vi "Temperature serial v7.vi"(0 "Command String":string, 5 "Time Out (S)":dbl, 7 "CALIB":dbl) -> (4 "T1":dbl, 6 "T2":dbl, 8 "T3":dbl, 10 "T4":dbl, 13 "error":bool, 14 "output cluster":cluster{dbl, dbl, dbl, dbl, i32, "error #":dbl}, 15 "Unit ID":dbl)   [LabVIEW 2017]
uses:
  Global 1.vi
panel:
  out "error out":errorcluster
  out "COM port":refnum<visa-resource-name>="COM6"
  out "error #":dbl
  out "End T":dbl
  out "Start T":dbl
  out "read time":dbl
  in  "Array - String":string[](array[string])
  out "end of data (#)":bool
  out "data bytes read":dbl
  out "data string":string
  out "read buffer":string
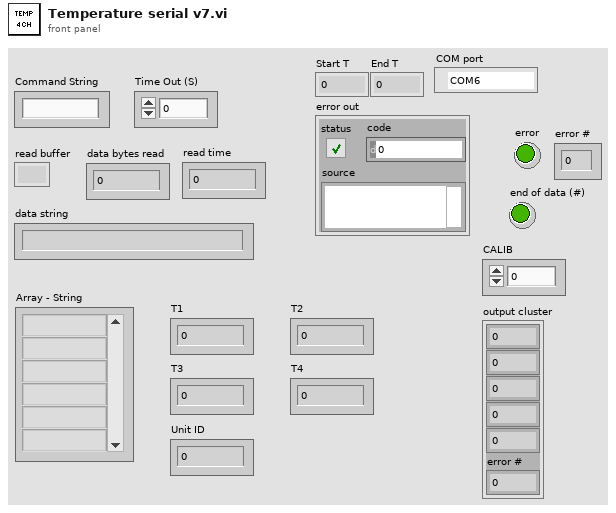
[diagram p1: front panel]
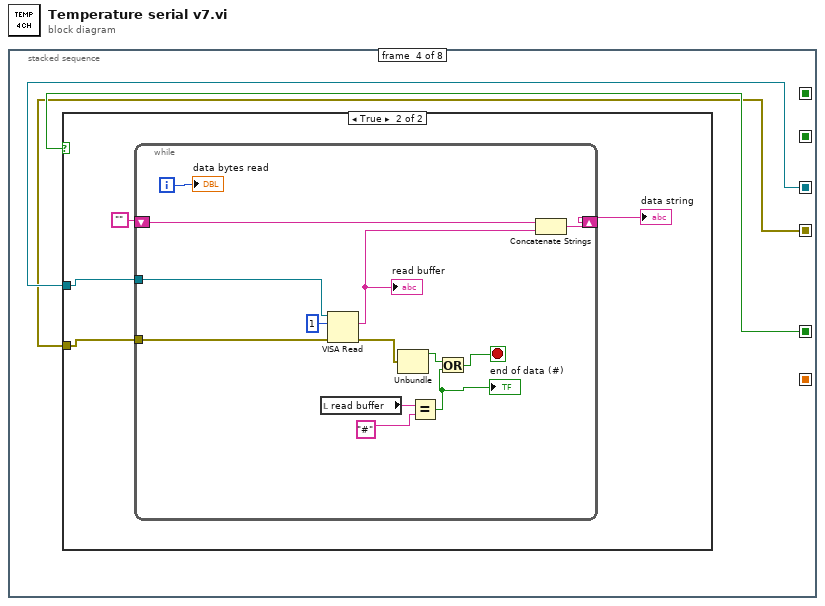
[diagram p0: block diagram]
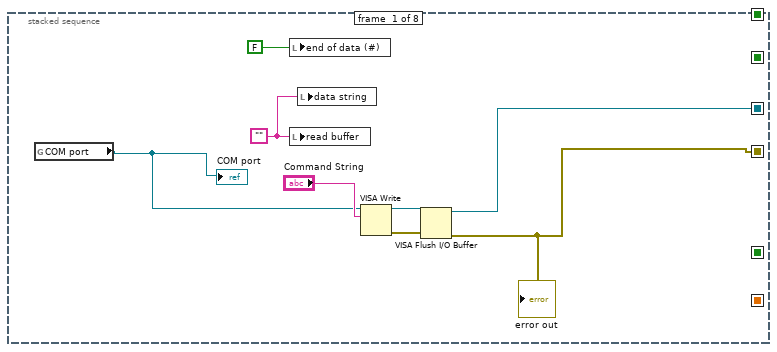
[diagram p2: hidden frame]
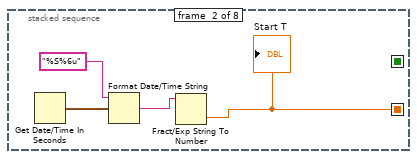
[diagram p3: hidden frame]
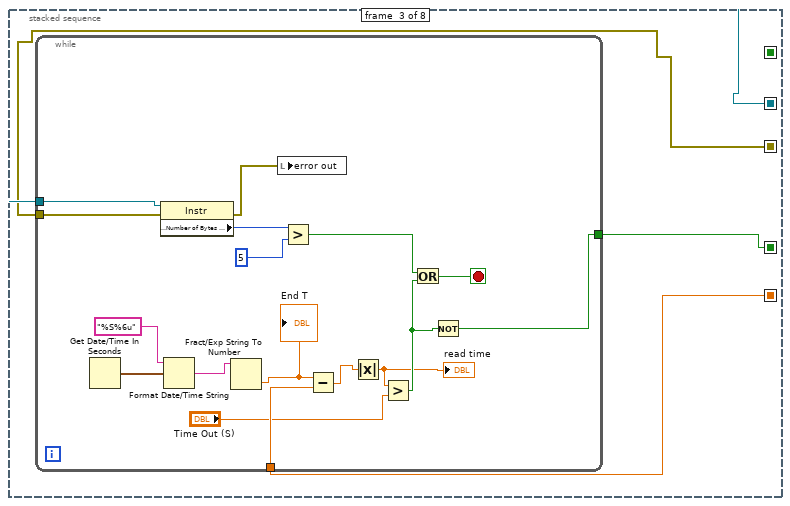
[diagram p4: hidden frame]
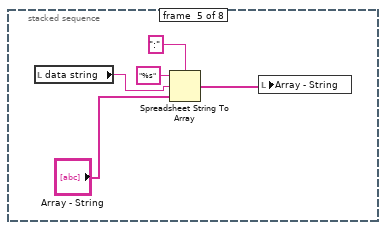
[diagram p6: hidden frame]
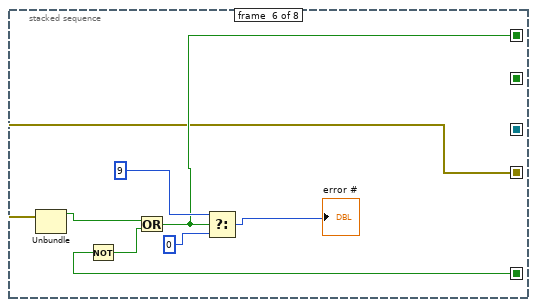
[diagram p7: hidden frame]
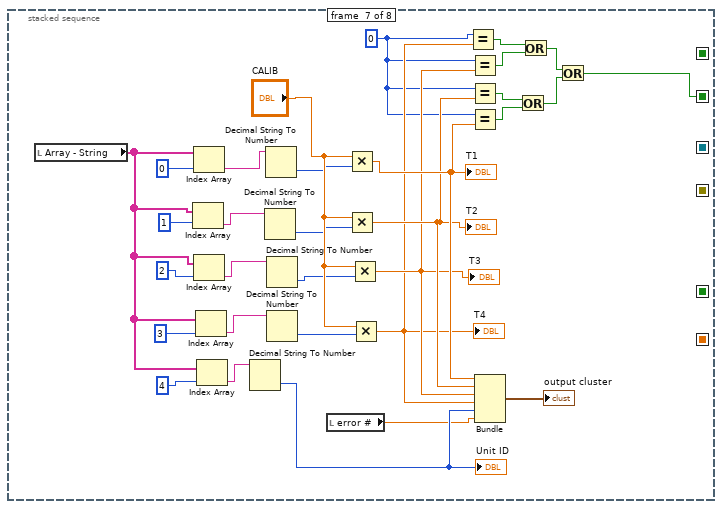
[diagram p8: hidden frame]
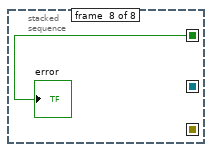
[diagram p9: hidden frame]
diagram:
  n1 = stacked-sequence {
    seq-local: [_ _ w16 _ _ _ _ _] -> [_ _ _ w36 _ w65 _ _]
    seq-local: [_ w9 _ _ _ _ _ _] -> [_ _ w15 _ _ _ _ _]
    seq-local: [_ _ _ _ _ w60 _ _] -> [_ _ _ _ _ _ _ _]
    seq-local: [_ _ _ _ _ _ w67 _] -> [_ _ _ _ _ _ _ w98]
    seq-local: [w2 _ _ _ _ _ _ _] -> [_ _ w14 w35 _ _ _ _]
    seq-local: [w1 _ _ _ _ _ _ _] -> [_ _ w13 w34 _ w59 _ _]
    frame #0 {
      w8 = ""
      n2 = global read "Global 1.vi" "COM port"() -> (w3:refnum<visa-resource-name>)
      "COM port" <- w3
      n3 = local write "end of data (#)"(FALSE) -> ()
      n4 = local write "read buffer"(w8) -> ()
      n5 = local write "data string"(w8) -> ()
      n6 = VISA Write(VISA resource name=w3, write buffer="Command String") -> (VISA resource name out=w5:refnum<visa-resource-name>, error out=w6:errorcluster)  [unwired: 1 in, 1 out]
      n7 = VISA Flush I/O Buffer(VISA resource name=w5, error in (no error)=w6) -> (VISA resource name out=w2:refnum<visa-resource-name>, error out=w1:errorcluster)  [unwired: 1 in]
      "error out" <- w1
    }
    frame #1 {
      n8 = Get Date/Time In Seconds() -> (seconds since 1Jan1904=w12:timestamp)
      n9 = Format Date/Time String(time format string (%c)="%S%6u", seconds (now)=w12) -> (date/time string=w10:string)  [unwired: 1 in]
      n10 = Fract/Exp String To Number(string=w10) -> (number=w9:dbl)  [unwired: 3 in, 1 out]
      "Start T" <- w9
    }
    frame #2 {
      n11 = while {
        tunnel: w14 -> [w33]
        tunnel: w13 -> [w32]
        tunnel: [w20] -> w16
        tunnel: w15 -> [w24]
        stop <- w22 stop-if-true
        n12 = Get Date/Time In Seconds() -> (seconds since 1Jan1904=w28:timestamp)
        n13 = property class="Instr"(reference=w33, error in=w32) -> (error out=w29:errorcluster, "Serial Settings:Number of Bytes at Serial Port"=w31:u32)  [unwired: 1 out]
        n14 = Format Date/Time String(time format string (%c)="%S%6u", seconds (now)=w28) -> (date/time string=w26:string)  [unwired: 1 in]
        n15 = Fract/Exp String To Number(string=w26) -> (number=w25:dbl)  [unwired: 3 in, 1 out]
        "End T" <- w25
        n16 = local write "error out"(w29) -> ()
        n17 = Greater?(x=w31, y=5) -> (0:w23:bool)
        n18 = Subtract(x=w25, y=w24) -> (x-y=w18:dbl)
        n19 = Absolute Value(x=w18) -> (abs(x)=w17:dbl)
        "read time" <- w17
        n20 = Greater?(x=w17, y="Time Out (S)") -> (0:w21:bool)
        n21 = Or(x=w23, y=w21) -> (x .or. y?=w22:bool)
        n22 = Not(x=w21) -> (.not. x?=w20:bool)
      }
    }
    frame #3 {
      n23 = case shown="True" w36 {
        tunnel: w35 -> [_ w40]
        tunnel: w34 -> [_ w39]
        frame False {
        }
        frame True {
          n24 = while {
            tunnel: w40 -> [w48]
            tunnel: w39 -> [w47]
            shift-right: [w46] -> w38
            shift-left: "" -> [w45]
            i -> [w49]
            stop <- w41 stop-if-true
            n25 = local read "read buffer"() -> (w52:string)
            n26 = VISA Read(VISA resource name=w48, byte count=u32 1, error in (no error)=w47) -> (read buffer=w50:string, error out=w44:errorcluster)  [unwired: 2 out]
            "read buffer" <- w50
            n27 = Unbundle(w44) -> ("status"=w43:bool)  [unwired: 2 out]
            n28 = Equal?(x=w52, y="#") -> (x = y?=w42:bool)
            "end of data (#)" <- w42
            n29 = Or(x=w43, y=w42) -> (x .or. y?=w41:bool)
            n30 = Concatenate Strings(w45, w50) -> (w46:string)
            "data bytes read" <- w49
          }
          "data string" <- w38
        }
      }
    }
    frame #4 {
      n31 = local read "data string"() -> (w56:string)
      n32 = Spreadsheet String To Array(delimiter (Tab)=":", format string="%s", spreadsheet string=w56, array type (2D Dbl)="Array - String") -> (array=w54:string[])
      n33 = local write "Array - String"(w54) -> ()
    }
    frame #5 {
      n34 = Unbundle(w59) -> ("status"=w66:bool)  [unwired: 2 out]
      n35 = Not(x=w65) -> (.not. x?=w64:bool)
      n36 = Or(x=w66, y=w64) -> (x .or. y?=w60:bool)
      n37 = Select(t=9, s=w60, f=0) -> (s? t:f=→"error #":i32)
    }
    frame #6 {
      w74 = 0
      n38 = local read "Array - String"() -> (w89:string[])
      n39 = Index Array(array=w89, index=1) -> (element=w92:string)
      n40 = Index Array(array=w89, index=0) -> (element=w96:string)
      n41 = Index Array(array=w89, index=2) -> (element=w91:string)
      n42 = Index Array(array=w89, index=3) -> (element=w90:string)
      n43 = Index Array(array=w89, index=4) -> (element=w87:string)
      n44 = Decimal String To Number(string=w87) -> (number=w81:i32)  [unwired: 2 in, 1 out]
      "Unit ID" <- w81
      n45 = Decimal String To Number(string=w92) -> (number=w84:i32)  [unwired: 2 in, 1 out]
      n46 = Decimal String To Number(string=w96) -> (number=w85:i32)  [unwired: 2 in, 1 out]
      n47 = Decimal String To Number(string=w91) -> (number=w83:i32)  [unwired: 2 in, 1 out]
      n48 = Decimal String To Number(string=w90) -> (number=w82:i32)  [unwired: 2 in, 1 out]
      n49 = local read "error #"() -> (w80:dbl)
      n50 = Multiply(x="CALIB", y=w85) -> (x*y=w78:dbl)
      "T1" <- w78
      n51 = Multiply(x="CALIB", y=w84) -> (x*y=w77:dbl)
      "T2" <- w77
      n52 = Multiply(x="CALIB", y=w83) -> (x*y=w76:dbl)
      "T3" <- w76
      n53 = Multiply(x="CALIB", y=w82) -> (x*y=w75:dbl)
      "T4" <- w75
      n54 = Equal?(x=w74, y=w75) -> (x = y?=w70:bool)
      n55 = Equal?(x=w74, y=w76) -> (x = y?=w71:bool)
      n56 = Equal?(x=w74, y=w77) -> (x = y?=w73:bool)
      n57 = Equal?(x=w74, y=w78) -> (x = y?=w72:bool)
      n58 = Bundle(w78, w77, w76, w75, w81, "error #"=w80) -> (→"output cluster":cluster{dbl, dbl, dbl, dbl, i32, "error #":dbl})  [unwired: 1 in]
      n59 = Or(x=w73, y=w72) -> (x .or. y?=w68:bool)
      n60 = Or(x=w70, y=w71) -> (x .or. y?=w69:bool)
      n61 = Or(x=w69, y=w68) -> (x .or. y?=w67:bool)
    }
    frame #7 {
      "error" <- w98
    }
  }
